vi "Configure Display.vi"(0 "VISA resource name":refnum<visa-resource-name>, 5 "Enable Display (True)":bool=TRUE, 7 "Enable Message Mode (False)":bool, 9 "Message (Empty)":string, 11 "error in (no error)":errorcluster) -> (4 "VISA resource name out":refnum<visa-resource-name>, 15 "error out":errorcluster)   [LabVIEW 2020, in "Keithley 27XX.lvlib"]
doc: "This VI controls the display on the front of the instrument."
uses:
  Keithley 27XX.lvlib
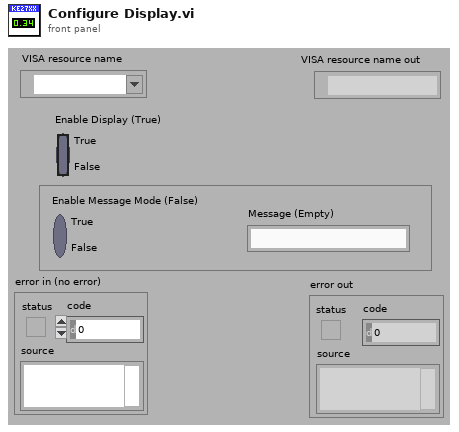
[diagram p1: front panel]
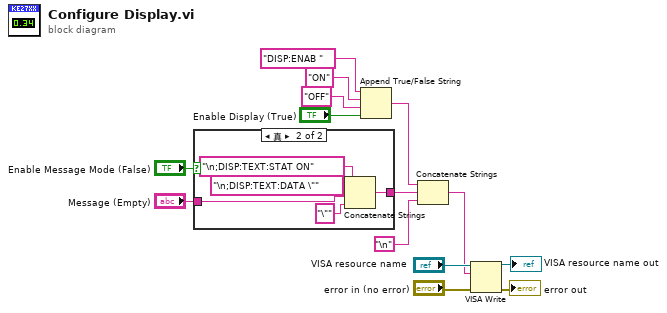
[diagram p0: block diagram]
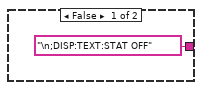
[diagram p2: hidden frame]
diagram:
  n1 = case shown="真" "Enable Message Mode (False)" {
    tunnel: "Message (Empty)" -> [_ w18]
    tunnel: ["\n;DISP:TEXT:STAT OFF" ("string (\"\")") w19] -> w4
    frame False {
    }
    frame True {
      n2 = Concatenate Strings("\n;DISP:TEXT:STAT ON" ("string (\"\")"), "\n;DISP:TEXT:DATA \"" ("string (\"\")"), w18, "\"" ("string")) -> (w19:string)
    }
  }
  n3 = Append True/False String(1:"Enable Display (True)", 2:"OFF" ("false string"), 3:"ON" ("true string"), 4:"DISP:ENAB " ("string (\"\")")) -> (0:w3:string)
  n4 = Concatenate Strings(w3, w4, "\n") -> (w2:string)
  n5 = VISA Write(VISA resource name="VISA resource name", write buffer=w2, error in (no error)="error in (no error)") -> (VISA resource name out=→"VISA resource name out":refnum<visa-resource-name>, error out=→"error out":errorcluster)  [unwired: 1 out]
